vi "getBubbleFeatures.vi"(0 "Image Src":T2, 1 "Range":cluster{"Lower value":sgl, "Upper value":sgl}={"Lower value"=128.0, "Upper value"=255.0} {"Upper value" format="%.2f"; "Lower value" format="%.2f"}, 2 "Operation":T1(ring), 5 "Min Radius":sgl=1.0 format="%.2f", 7 "Number of iterations (1)":i32=5, 8 "Number of iterations (1) 2":i32=5, 9 "Max Radius":sgl=10.0 format="%.2f", 11 "error in (no error)":errorcluster, 12 "Operation 2":T1(ring)) -> (3 "Image Dst Out 2":T2, 4 "Image Dst Out":T2, 6 "Circles Data":T3(array[cluster]), 10 "bubbleFeatures":T4, 13 "Plot SD":dbl(graph), 14 "Plot mean":dbl(graph), 15 "error out":errorcluster)   [LabVIEW 2013]
uses:
  <vilib>/vision/Image Controls.llb/IMAQ Image.ctl
  <vilib>/vision/NI_Vision_Development_Module.lvlib
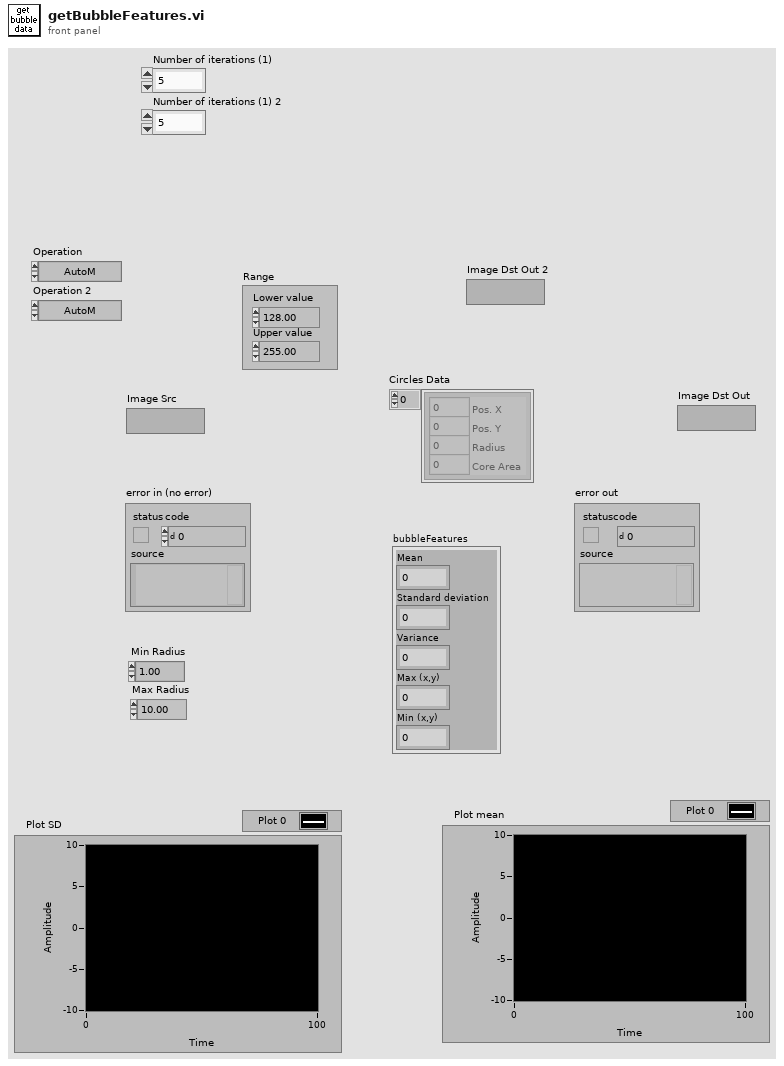
[diagram p1: front panel]
types:
  T1 = enum32{"AutoM", "Close", "Dilate", "Erode", "Gradient", "Gradient out", "Gradient in", "Hit miss", "Open", "PClose", "POpen", "Thick", "Thin"}
  T2 = typedef "IMAQ Image.ctl" = refnum<image>
  T3 = cluster{"Pos. X":i32, "Pos. Y":i32, "Radius":i32, "Core Area":i32}[]
  T4 = cluster{"Mean":dbl, "Standard deviation":dbl, "Variance":dbl, "Max (x,y)":dbl, "Min (x,y)":dbl}
  T5 = typedef "Image Type" = u32
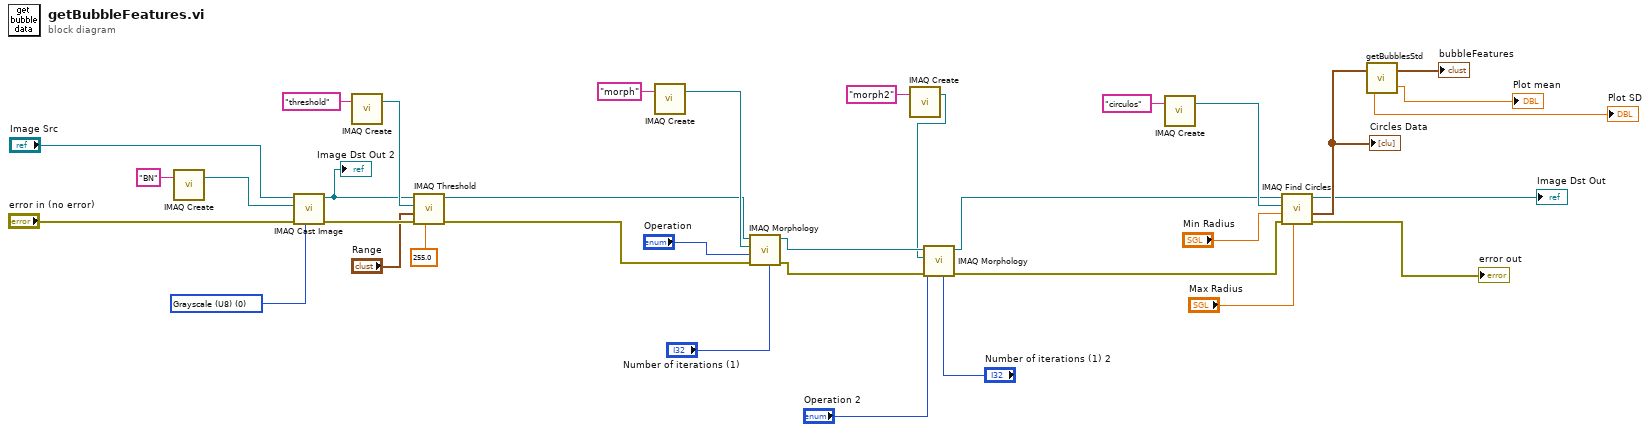
[diagram p0: block diagram]
diagram:
  w24 = T5 0 items=["Grayscale (U8)", "Grayscale (I16)", "Grayscale (SGL)", "Complex (CSG)", "RGB (U32)", "HSL (U32)", "RGB (U64)", "Grayscale (U16)"] ("Image Type")
  n1 = call "IMAQ Create"("Image Name"="BN") -> ("New Image"=w35:T2)  [unwired: 4 in, 1 out]
  n2 = call "IMAQ Cast Image"("Image Type"=w24, "error in (no error)"="error in (no error)", "Image Dst"=w35, "Image Src"="Image Src") -> ("error out"=w32:errorcluster, "Image Dst Out"=w17:T2)  [unwired: 6 in]
  "Image Dst Out 2" <- w17
  n3 = call "IMAQ Create"("Image Name"="threshold") -> ("New Image"=w30:T2)  [unwired: 4 in, 1 out]
  n4 = call "IMAQ Threshold"("Replace Value"=sgl 255.0, "error in (no error)"=w32, "Range"="Range", "Image Dst"=w30, "Image Src"=w17) -> ("error out"=w7:errorcluster, "Image Dst Out"=w11:T2)  [unwired: 5 in]
  n5 = call "IMAQ Create"("Image Name"="morph") -> ("New Image"=w12:T2)  [unwired: 4 in, 1 out]
  n6 = call "IMAQ Morphology"("Number of iterations (1)"="Number of iterations (1)", "error in (no error)"=w7, "Operation"="Operation", "Image Dst"=w12, "Image Src"=w11) -> ("error out"=w6:errorcluster, "Image Dst Out"=w10:T2)  [unwired: 5 in]
  n7 = call "IMAQ Create"("Image Name"="morph2") -> ("New Image"=w9:T2)  [unwired: 4 in, 1 out]
  n8 = call "IMAQ Morphology"("Number of iterations (1)"="Number of iterations (1) 2", "error in (no error)"=w6, "Operation"="Operation 2", "Image Dst"=w9, "Image Src"=w10) -> ("error out"=w5:errorcluster, "Image Dst Out"=w8:T2)  [unwired: 5 in]
  n9 = call "IMAQ Create"("Image Name"="circulos") -> ("New Image"=w27:T2)  [unwired: 4 in, 1 out]
  n10 = call "IMAQ Find Circles"("Max Radius"="Max Radius", "error in (no error)"=w5, "Min Radius"="Min Radius", "Image Dst"=w27, "Image Src"=w8) -> ("error out"=→"error out":errorcluster, "Circles Data"=w21:T3, "Image Dst Out"=→"Image Dst Out":T2)  [unwired: 3 in, 1 out]
  "Circles Data" <- w21
  n11 = call "getBubblesStd.vi"("Circles Data in"=w21) -> ("Plot mean"=→"Plot mean":dbl, "bubbleFeatures"=→"bubbleFeatures":T4, "Plot SD"=→"Plot SD":dbl)
